vi "TEST_A3FPort-Steffen’s MacBook Pro.vi"() -> ()   [LabVIEW 2018]
uses:
  <vilib>/myRIO/Common/Instrument Driver Framework/myRIO v1.0/UART/vis/myRIO v1.0 Close UART.vi
  <vilib>/Utility/error.llb/Error Cluster From Error Code.vi
  <vilib>/myRIO/Common/Instrument Driver Framework/myRIO v1.0/DIO/vis/myRIO v1.0 Write DIO.vi
  <vilib>/myRIO/Common/Instrument Driver Framework/Utilities/vis/FPGA Ref Manager.vi
  <vilib>/myRIO/Common/Instrument Driver Framework/myRIO v1.0/myRIO v1.0 Reset FPGA.vi
  <vilib>/myRIO/Common/Instrument Driver Framework/myRIO v1.0/IRQ/vis/myRIO v1.0 IRQ Info FGV.vi
  <vilib>/myRIO/Common/Instrument Driver Framework/myRIO v1.0/IRQ/vis/myRIO v1.0 Timer IRQ Info FGV.vi
  <vilib>/myRIO/Common/Instrument Driver Framework/myRIO v1.0/IRQ/vis/myRIO v1.0 ISR Agent.vi
  <vilib>/myRIO/Instrument Drivers/Utilities/Utilities.lvlib
  <vilib>/myRIO/Instrument Drivers/Onboard IO/DIO/DIO.lvlib
panel:
  out "Value out":dbl
  in  "Enum":enum16{"F3", "F4", "F5", "F6", "F7", "F8"}(ring)
  in  "stop":bool
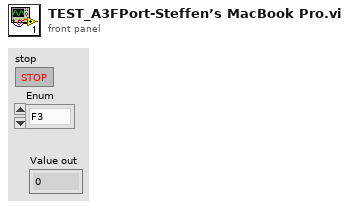
[diagram p1: front panel]
types:
  T1 = typedef "DIO.lvlib/DIO Reference.ctl" = cluster{"myRIO Reference":T2, "DIO Channels List":T6}
  T2 = typedef "myRIO Generic Hardware Reference.ctl" = cluster{"myRIO Model":T3, "myRIO Hardware Reference":T4}
  T3 = typedef "Hardware Version Enum.ctl" = enum16{"Unknown", "myRIO-1900", "myRIO-1950", "roboRIO", "NI ELVIS RIO CM", "ELVIS III"}
  T4 = typedef "myRIO v1.0 Reference.ctl" = cluster{"Generic FPGA Reference":T5, "Allow multiple opens":bool}
  T5 = typedef "Generic FPGA Reference.ctl" = refnum<k20>
  T6 = typedef "DIO Channels List.ctl" = T7[]
  T7 = typedef "DIO Channels Enum.ctl" = enum16{"Not Connected", "C/DIO0", "C/DIO1", "C/DIO2", "C/DIO3", "C/DIO4", "C/DIO5", "C/DIO6", "C/DIO7", "A/DIO0", "A/DIO1", "A/DIO2", "A/DIO3", "A/DIO4", "A/DIO5", "A/DIO6", "A/DIO7", "A/DIO8", "A/DIO9", "A/DIO10", "A/DIO11", "A/DIO12", "A/DIO13", "A/DIO14", "A/DIO15", "A/DIO16", "A/DIO17", "A/DIO18", "A/DIO19", "B/DIO0", "B/DIO1", "B/DIO2", "B/DIO3", "B/DIO4", "B/DIO5", "B/DIO6", "B/DIO7", "B/DIO8", "B/DIO9", "B/DIO10", "B/DIO11", "B/DIO12", "B/DIO13", "B/DIO14", "B/DIO15", "B/DIO16", "B/DIO17", "B/DIO18", "B/DIO19", "LED0", "LED1", "LED2", "LED3", "Button0", "DIO/DIO0", "DIO/DIO1", "DIO/DIO2", "DIO/DIO3", "DIO/DIO4", "DIO/DIO5", "DIO/DIO6", "DIO/DIO7", "DIO/DIO8", "DIO/DIO9", "SPI/CS0", "SPI/CS1", "SPI/CS2", "SPI/CS3", "LED RADIO (Green)", "LED RADIO (Red)", "LED COMM (Green)", "LED COMM (Red)", "LED MODE (Green)", "LED MODE (Red)"}
  T8 = typedef "PWM.lvlib/PWM Reference.ctl" = cluster{"myRIO Reference":T2, "PWM Channels Enum":T9, "PWM Configuration":T10}
  T9 = typedef "PWM Channels Enum.ctl" = enum16{"Not Connected", "C/PWM0", "C/PWM1", "A/PWM0", "A/PWM1", "A/PWM2", "A/PWM3", "A/PWM4", "A/PWM5", "A/PWM6", "A/PWM7", "A/PWM8", "A/PWM9", "A/PWM10", "A/PWM11", "A/PWM12", "A/PWM13", "A/PWM14", "A/PWM15", "A/PWM16", "A/PWM17", "A/PWM18", "A/PWM19", "B/PWM0", "B/PWM1", "B/PWM2", "B/PWM3", "B/PWM4", "B/PWM5", "B/PWM6", "B/PWM7", "B/PWM8", "B/PWM9", "B/PWM10", "B/PWM11", "B/PWM12", "B/PWM13", "B/PWM14", "B/PWM15", "B/PWM16", "B/PWM17", "B/PWM18", "B/PWM19", "PWM/PWM0", "PWM/PWM1", "PWM/PWM2", "PWM/PWM3", "PWM/PWM4", "PWM/PWM5", "PWM/PWM6", "PWM/PWM7", "PWM/PWM8", "PWM/PWM9"}
  T10 = typedef "PWM.lvlib/PWM Configuration.ctl" = cluster{"Frequency":dbl, "Duty Cycle":dbl}
  T11 = typedef "Accelerometer.lvlib/Accelerometer Reference.ctl" = cluster{"myRIO Reference":T2, "Accelerometer Channels List":T12, "LSB Weight":dbl}
  T12 = typedef "Accelerometer Channels List.ctl" = T13[]
  T13 = typedef "Accelerometer Channels Enum.ctl" = enum16{"Not Connected", "X-Axis", "Y-Axis", "Z-Axis"}
  T14 = typedef "AI.lvlib/AI Reference.ctl" = cluster{"myRIO Reference":T2, "AI Channels List":T15, "AI Scaling Constants List":T17}
  T15 = typedef "AI Channels List.ctl" = T16[]
  T16 = typedef "AI Channels Enum.ctl" = enum16{"Not Connected", "AudioIn/Left", "AudioIn/Right", "C/AI0", "C/AI1", "A/AI0", "A/AI1", "A/AI2", "A/AI3", "A/AI4", "A/AI5", "A/AI6", "A/AI7", "B/AI0", "B/AI1", "B/AI2", "B/AI3", "B/AI4", "B/AI5", "B/AI6", "B/AI7", "AI/AI0", "AI/AI1", "AI/AI2", "AI/AI3", "A/AI0 (DIFF)", "A/AI1 (DIFF)", "A/AI2 (DIFF)", "A/AI3 (DIFF)", "B/AI0 (DIFF)", "B/AI1 (DIFF)", "B/AI2 (DIFF)", "B/AI3 (DIFF)"}
  T17 = typedef "Analog Scaling Constants List.ctl" = T18[]
  T18 = typedef "Analog Scaling Constants.ctl" = cluster{"LSB Weight (Volts)":dbl, "Offset (Volts)":dbl, "Signed?":bool}
  T19 = typedef "SPI.lvlib/SPI Reference.ctl" = cluster{"myRIO Reference":T2, "SPI Channels Enum":T20, "SPI Configuration":T21}
  T20 = typedef "SPI Channels Enum.ctl" = enum16{"Not Connected", "A/SPI", "B/SPI", "SPI/SPI"}
  T21 = typedef "SPI.lvlib/SPI Configuration.ctl" = cluster{"Frequency [Hz]":dbl, "Clock Phase":T22, "Clock Polarity":T23, "Data Direction":T24, "Frame Length":T25}
  T22 = typedef "SPI Clock Phase.ctl" = enum8{"Leading", "Trailing"}
  T23 = typedef "SPI Clock Polarity.ctl" = enum8{"Low", "High"}
  T24 = typedef "SPI Data Direction.ctl" = enum8{"Most significant bit first", "Least significant bit first"}
  T25 = typedef "SPI Frame Length.ctl" = u8
  T26 = cluster{"B/DIO0 - Stepper Direction":T1, "B/DIO1 - Stepper1 Enable":T1, "B/DIO2 - Stepper2 Enable":T1, "B/DIO3 - Stepper3 Enable":T1, "B/DIO4 - Endstop Stepper1 Top":T1, "B/DIO11 - Endstop Stepper1 Bund":T1, "B/DIO12 - Endstop Stepper2 Top":T1, "B/DIO13 - Endstop Stepper2 Bund":T1, "B/DIO14 - Endstop Stepper3 Top":T1, "B/DIO15 - Endstop Stepper3 Bund":T1, "A/DIO0 - Cooler":T1, "A/DIO1 - Beacon drop (dio1)":T1, "A/DIO2 - Beacon drop (dio0)":T1, "A/DIO3 - QuickRelease (dio1)":T1, "A/DIO4 - QuickRelease (dio0)":T1, "A/DIO11 - LiDAR SPI CS":T1, "B/PWM0 - Stepper":T8, "B/PWM1 - Drill":T8, "A/PWM0 - Servo_Roll":T8, "A/PWM1 - Servo_Yaw":T8, "Acc. X-axis":T11, "Acc. Y-axis":T11, "B/AI0 - Drone Grounded S1 - F3":T14, "A/AI0 - QuickRelease S4 - F4":T14, "B/AI2 - Beacon Drop S5 - F5":T14, "B/AI3 - Begin drilling S3 - F6":T14, "B/AI1 - Gimbal Seach S8 - F8":T14, "A/AI1 - Beacon Wiper":T14, "A/AI2 - QuickRelease Wiper":T14, "A/AI3 - Drill Current":T14, "A/SPI - LiDAR":T19, "B/UART - XBee":refnum<visa-resource-name>, "A/UART - A3 GPS":refnum<visa-resource-name>, "RIO Flashing LEDs":T1}
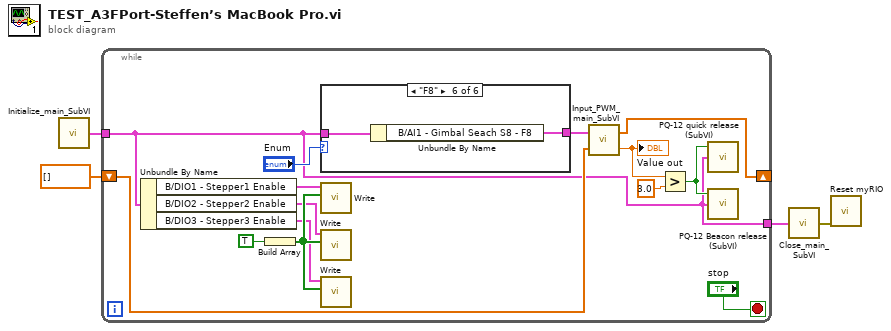
[diagram p0: block diagram]
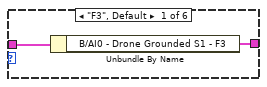
[diagram p2: hidden frame]
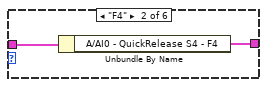
[diagram p3: hidden frame]
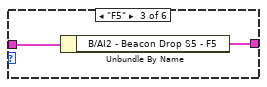
[diagram p4: hidden frame]
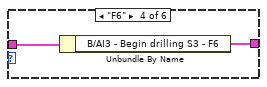
[diagram p5: hidden frame]
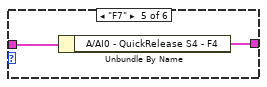
[diagram p6: hidden frame]
diagram:
  n1 = call "Initialize_main_SubVI.vi"() -> ("output cluster"=w4:T26)
  n2 = while {
    tunnel: w4 -> [w5]
    tunnel: [w5] -> w2
    shift-right: [w16] -> _
    shift-left: dbl[] [] ("Shift out") -> [w15]
    stop <- "stop" stop-if-true
    n3 = Unbundle By Name(w5) -> ("B/DIO1 - Stepper1 Enable"=w12:T1, "B/DIO2 - Stepper2 Enable"=w11:T1, "B/DIO3 - Stepper3 Enable"=w10:T1)
    n4 = Build Array(TRUE) -> (w13:bool[])
    n5 = case shown="\"F8\"" "Enum" {
      tunnel: w5 -> [w20 w22 w24 w26 w28 w30]
      tunnel: [w19 w21 w23 w25 w27 w29] -> w9
      frame "F3", Default {
        n6 = Unbundle By Name(w20) -> ("B/AI0 - Drone Grounded S1 - F3"=w19:T14)
      }
      frame "F4" {
        n7 = Unbundle By Name(w22) -> ("A/AI0 - QuickRelease S4 - F4"=w21:T14)
      }
      frame "F5" {
        n8 = Unbundle By Name(w24) -> ("B/AI2 - Beacon Drop S5 - F5"=w23:T14)
      }
      frame "F6" {
        n9 = Unbundle By Name(w26) -> ("B/AI3 - Begin drilling S3 - F6"=w25:T14)
      }
      frame "F7" {
        n10 = Unbundle By Name(w28) -> ("A/AI0 - QuickRelease S4 - F4"=w27:T14)
      }
      frame "F8" {
        n11 = Unbundle By Name(w30) -> ("B/AI1 - Gimbal Seach S8 - F8"=w29:T14)
      }
    }
    n12 = call <vilib>:"Write.vi"("Values"=w13, "DIO Ref In"=w12) -> ()  [unwired: 7 in, 2 out]
    n13 = call <vilib>:"Write.vi"("Values"=w13, "DIO Ref In"=w11) -> ()  [unwired: 7 in, 2 out]
    n14 = call <vilib>:"Write.vi"("Values"=w13, "DIO Ref In"=w10) -> ()  [unwired: 7 in, 2 out]
    n15 = call "Input_PWM_main_SubVI.vi"("Shift in"=w15, "AI Ref In"=w9) -> ("Value out"=w8:dbl, "Shift out"=w16:dbl[])
    "Value out" <- w8
    n16 = Greater?(x=w8, y=3.0) -> (0:w6:bool)
    n17 = call "PQ-12 quick release (SubVI).vi"("output cluster"=w5, "Extend / Retract [F/T]"=w6) -> ()  [unwired: 1 in, 1 out]
    n18 = call "PQ-12 Beacon release (SubVI).vi"("output cluster"=w5, "Extend / Retract [T/F]"=w6) -> ()  [unwired: 1 in, 1 out]
  }
  n19 = call "Close_main_SubVI.vi"("output cluster"=w2) -> ("error constant"=w3:errorcluster)
  n20 = call <vilib>:"Reset myRIO.vi"("error in (no error)"=w3) -> ()  [unwired: 10 in, 1 out]
